vi "D3DM_comm.vi"() -> ()   [LabVIEW 2013]
uses:
  <vilib>/Native 3D Graph/xcontrol/3DPC_SurfacePlot.xctl
  <vilib>/Platform/NI_3dgraph.lvlib
panel:
  out "InRange":bool
  in  "3D Curve - Lorenz Attractor":refnum<k7>(container)
  in  "Simulation":bool
  in  "Least Dis":dbl=200.0
  in  "holder_length":dbl=87.37
  in  "Arm Angle Set":i32(slide)=1456 min=750 max=2150 step=1 scale=750.0..2150.0
  out "Title":string="      Distributed 3D Measurement Control Panel"
  in  "Log File Path":path=path "E:/Dropbox/StaredProject/Distributed3D/D3DM/raw_log.txt"
  in  "Port":u16=8899
  in  "Base Rotation Speed Set":i32(slide)=1471 min=1000 max=2000 step=1 scale=1000.0..2000.0
  in  "Command":string
  in  "Byte to Read(TCP)":i32=512
  out "Read Buffer":string
  out "help":string="1.Set the target Port number;\n2.Press \"Ready\" button to start acquiring data;\n3.Use arrow keys to control movement;\n4.Use the speed pointer slide to control speed;\n5.Use the Arm Angle slide to control arm;\n6.Press \"ESC\" to stop the car, 3D plot should be     finished automatically."
  in  "ArcStepThreshold":dbl=8000.0
  out "3D Graph":refnum<class "Base Datatype.lvclass">[](xcontrol)
  in  "Stop Button":bool
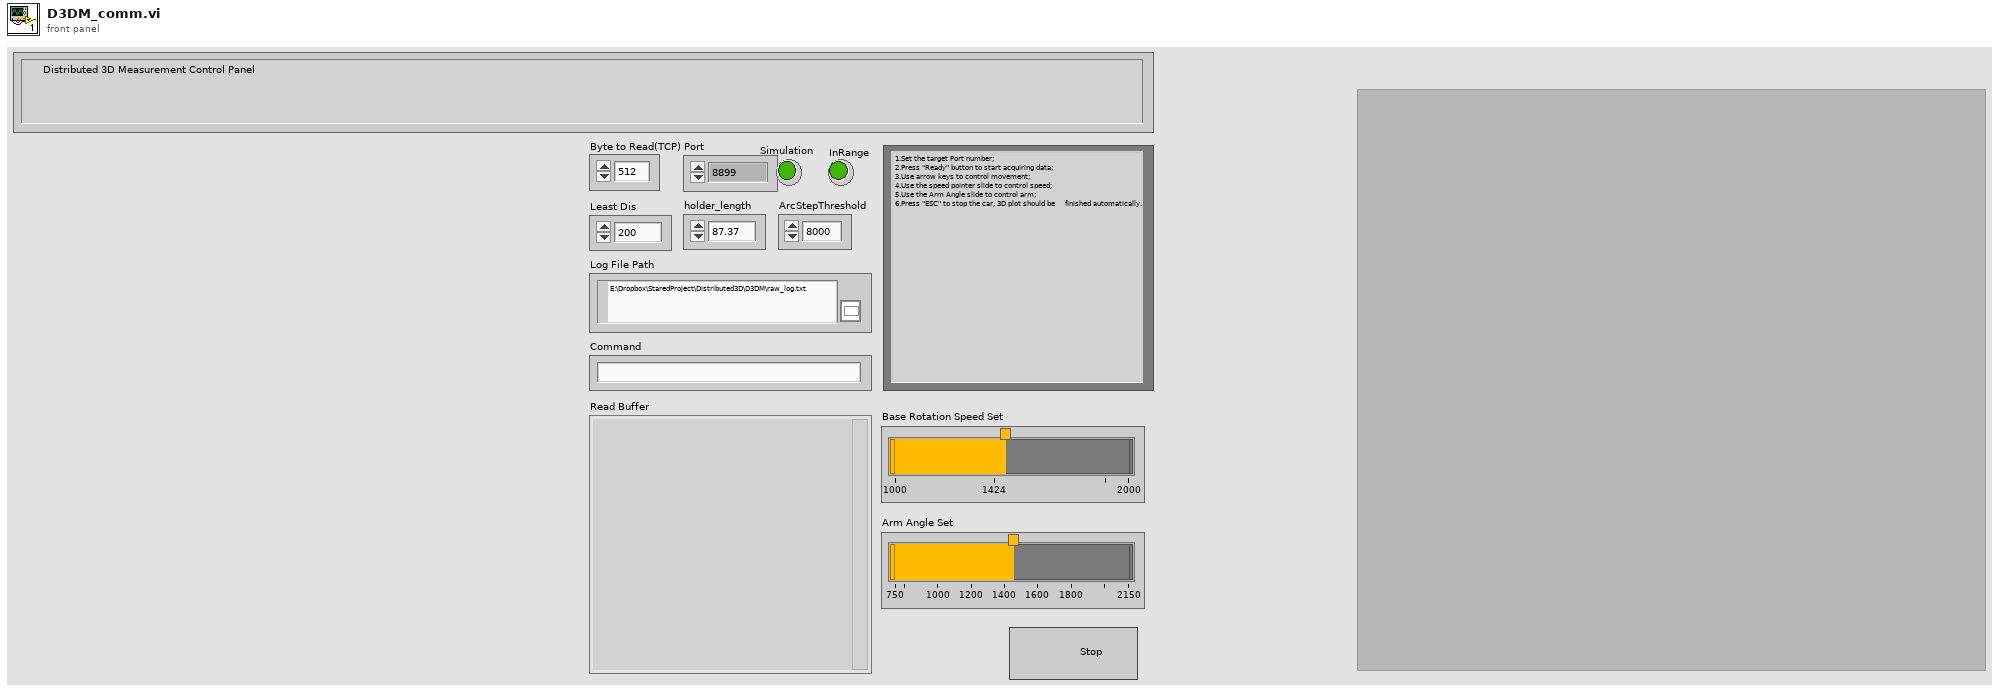
[diagram p1: front panel]
types:
  T1 = enum16{"open", "replace", "create", "open or create", "replace or create", "replace or create with confirmation"}
  T2 = typedef "eventvkey.ctl" = enum16{"ASCII", "Enter", "Return", "Shift", "Ctrl", "Alt", "Cmd", "Opt", "Caps", "NumLock", "Clear", "Break", "Up", "Down", "Left", "Right", "Insert", "Delete", "Home", "End", "PageUp", "PageDown", "Escape", "Help", "Pause", "ScrollLock", "F1", "F2", "F3", "F4", "F5", "F6", "F7", "F8", "F9", "F10", "F11", "F12", "F13", "F14", "F15", "F16", "F17", "F18", "F19", "F20", "F21", "F22", "F23", "F24", "Play", "VolumeUp", "VolumeDown", "Mute", "Two Byte Char"}
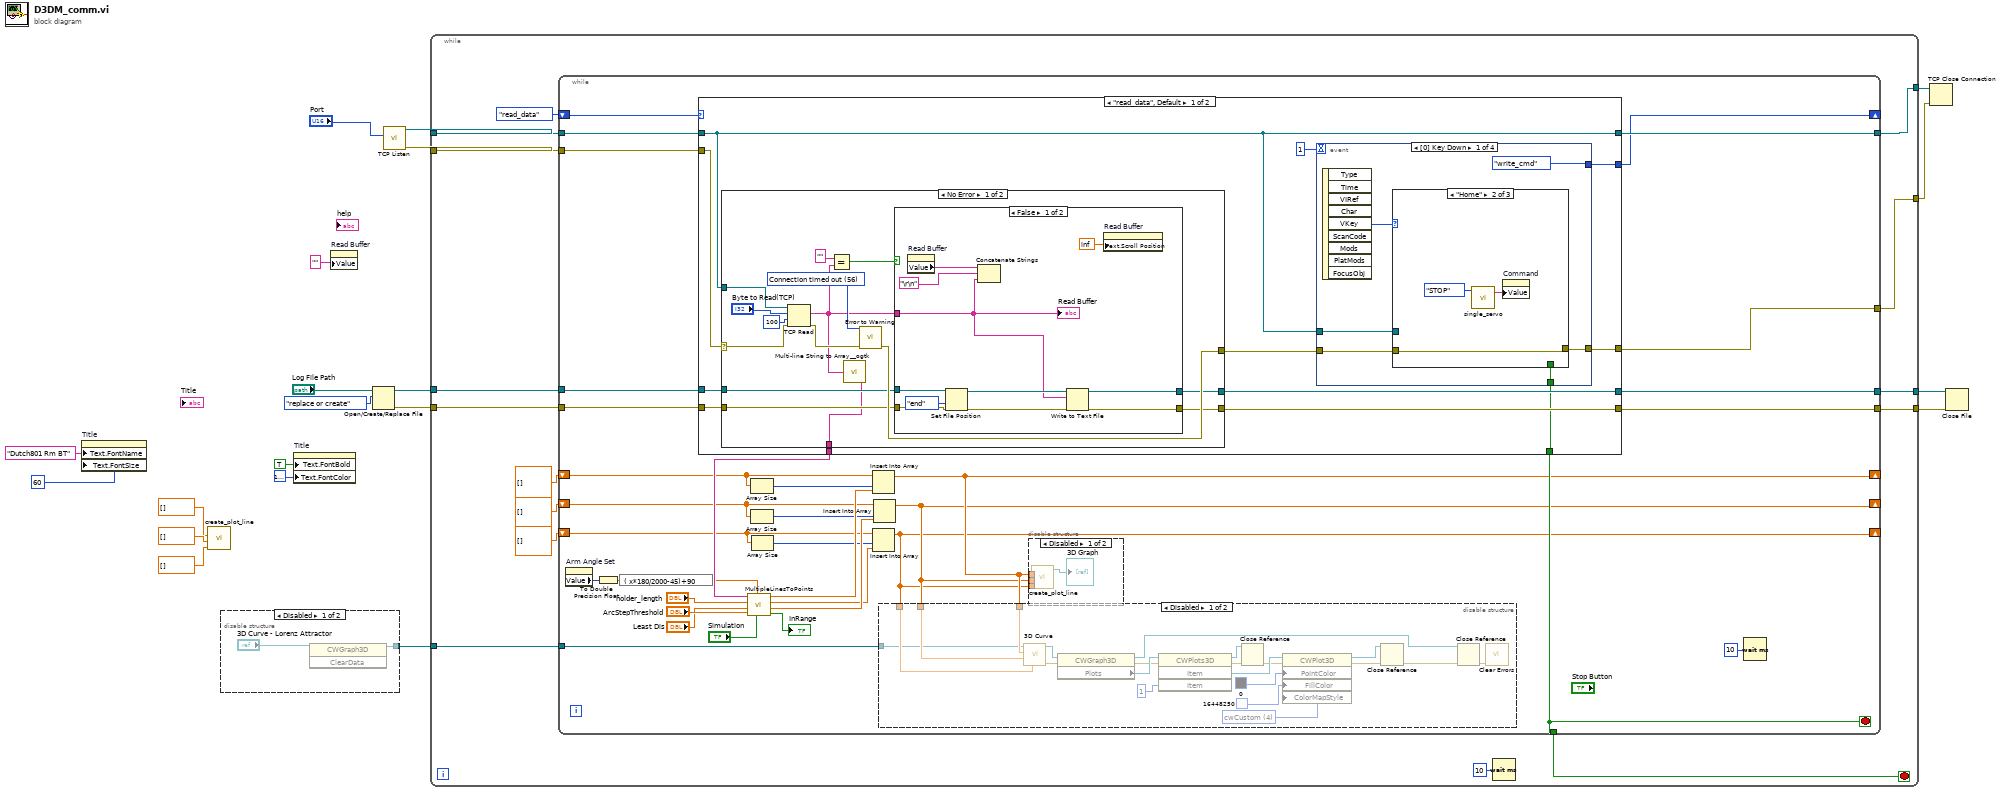
[diagram p0: block diagram]
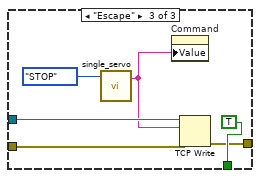
[diagram p6: hidden frame]
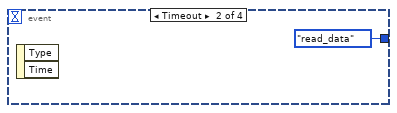
[diagram p7: hidden frame]
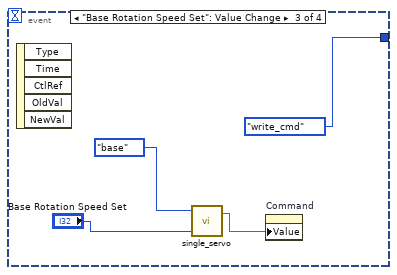
[diagram p8: hidden frame]
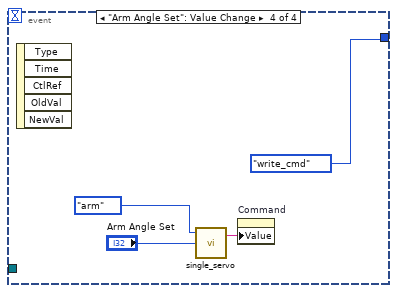
[diagram p9: hidden frame]
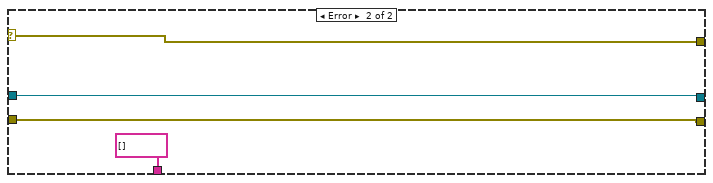
[diagram p11: hidden frame]
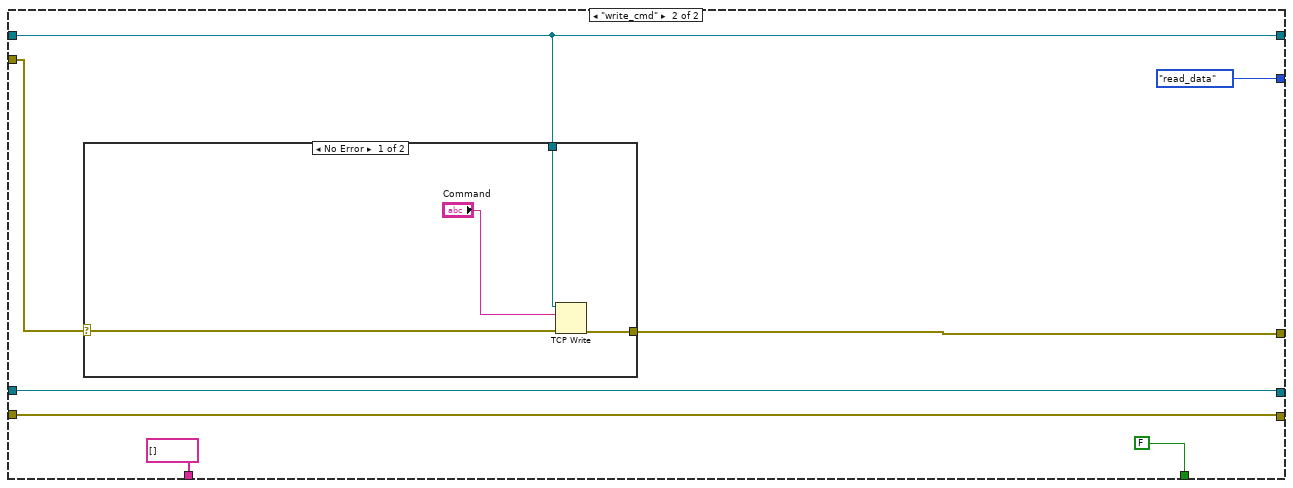
[diagram p12: hidden frame]
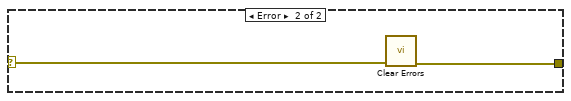
[diagram p13: hidden frame]
diagram:
  n1 = property on="Title" class="Str"("Text.FontName"="Dutch801 Rm BT" ("Text.Font:Name"), "Text.FontSize"=u32 60 ("Text.Font:Size")) -> ()  [unwired: 2 in, 2 out]
  n2 = call <vilib>:"create_plot_line.vi"("z vector"=dbl[] [], "y vector"=dbl[] [], "x vector"=dbl[] []) -> ()  [unwired: 8 in, 1 out]
  n3 = disable-structure shown="Disabled" {
    disable-tunnel: [w21 _] -> w1
    frame Disabled {
      n4 = invoke class="CWGraph3D" method="ClearData"(reference="3D Curve - Lorenz Attractor") -> (reference out=w21:refnum<k7>)  [unwired: 2 in, 2 out]
    }
    frame Enabled {
    }
  }
  n5 = property on="Title" class="Str"("Text.FontBold"=TRUE ("Text.Font:Bold"), "Text.FontColor"=u32 16777222) -> ()  [unwired: 2 in, 2 out]
  n6 = property on="Read Buffer" class="Str"("Value"="") -> ()  [unwired: 2 in, 2 out]
  n7 = Open/Create/Replace File(file path (use dialog)="Log File Path", operation (0:open)=T1."replace or create") -> (refnum out=w13:refnum<file>, error out=w12:errorcluster)  [unwired: 4 in, 1 out]
  n8 = call <vilib>:"TCP Listen.vi"("port"="Port") -> ("error out"=w18:errorcluster, "connection ID"=w19:refnum<k5>)  [unwired: 6 in, 3 out]
  n9 = while {
    tunnel: w19 -> [w35]
    tunnel: w18 -> [w34]
    tunnel: [w33] -> w17
    tunnel: [w32] -> w16
    tunnel: w13 -> [w31]
    tunnel: w12 -> [w30]
    tunnel: [w29] -> w11
    tunnel: [w28] -> w10
    tunnel: w1 -> [w27]
    stop <- w36 stop-if-true
    n10 = while {
      shift-right: [w61] -> _
      shift-left: enum16{"read_data", "write_cmd"}."read_data" ("RWstate") -> [w71]
      tunnel: w34 -> [w70]
      tunnel: w35 -> [w69]
      tunnel: [w64] -> w36
      tunnel: w31 -> [w68]
      tunnel: w30 -> [w67]
      tunnel: [w66] -> w29
      tunnel: [w65] -> w28
      tunnel: [w63] -> w33
      tunnel: [w62] -> w32
      shift-right: [w49] -> _
      shift-left: dbl[] [] -> [w56]
      shift-right: [w48] -> _
      shift-left: dbl[] [] -> [w52]
      shift-right: [w47] -> _
      shift-left: dbl[] [] -> [w51]
      tunnel: w27 -> [w43]
      stop <- w64 stop-if-true
      n11 = property on="Arm Angle Set" class="Slide (strict)"() -> ("Value"=w41:i32)  [unwired: 2 in, 2 out]
      n12 = To Double Precision Float(number=w41) -> (double precision float=w39:dbl)
      n13 = expression code="( x*180/2000-45)+90"(w39) -> (w40:dbl)
      n14 = case shown="\"read_data\", Default" w71 {
        tunnel: w70 -> [w108 w173]
        tunnel: w69 -> [w100 w168]
        tunnel: w68 -> [w107 w172]
        tunnel: w67 -> [w106 w171]
        tunnel: [w105 w172] -> w66
        tunnel: [w104 w171] -> w65
        tunnel: [w103 FALSE] -> w64
        tunnel: [w101 w170] -> w63
        tunnel: [w100 w168] -> w62
        tunnel: [w99 enum16{"read_data", "write_cmd"}."read_data" ("RWstate")] -> w61
        tunnel: [w97 string[] [] ("lines")] -> w57
        frame "read_data", Default {
          n15 = case shown="No Error" w108 {
            selector: w108 -> [w140 w165]
            tunnel: [w144 w165] -> w102
            tunnel: w100 -> [w141 _]
            tunnel: w107 -> [w139 w164]
            tunnel: w106 -> [w138 w163]
            tunnel: [w137 w164] -> w105
            tunnel: [w136 w163] -> w104
            tunnel: [w134 string[] [] ("lines")] -> w97
            frame No Error {
              w148 = 56 items=["No Error", "Argument Error", "Memory Full", "Out of Zone", "End of File", "File Already Open", "Generic File IO Error", "File Not Found", "File Permission Error", "Disk Full", "Duplicate Path", "Too Many Files Open", "Not Enabled", "Resource File Not Found", "Cannot Add Resource", "Resource Not Found", "Image Not Found", "Image Memory Error", "Pen Does Not Exist", "Config Bad Type", "Config Token Not Found", "Config Parse Error", "Config Memory Error", "Bad External Code Format", "Bad External Code Offset", "External Code Not Present", "Null Window", "Destroy Window Mixup", "Null Menu", "Print Aborted", "Bad Print Record", "Print Driver Error", "Windows Error During Print", "Memory Error During Print", "Print Dialog Error", "Generic Print Error", "Invalid Device Refnum", "Device Not Found", "Device Parameter Error", "Device Unit Error", "Can't Open Device", "Device Call Aborted", "Generic Error", "Cancelled By User", "Object ID Too Low", "Object ID Too High", "Object Not In Heap", "Unknown Heap", "Bad DefProc ID", "DefProc Not In Table", "Message Out Of Range", "Null Method", "Unknown Message", "Manager Call Not Supported", "Bad address", "Connection In progress", "Connection timed out", "Connection is already in progress", "Network attribute not supported", "Network error", "Address in use", "System out of memory", "Connection aborted", "Connection refused", "Connection is not connected", "Connection is already connected", "Connection closed", "Initialize error (interapplication manager)", "Bad occurrence", "Wait on unbound occurrence handler", "Occurrence queue overflow", "Bad path", "Semaphore not signaled", "Unrecognized type (interapplication manager)"] ("1st Error to Convert")
              n16 = TCP Read(connection ID=w141, bytes to read="Byte to Read(TCP)", error in (no error)=w140, 9:100) -> (data out=w135:string, error out=w147:errorcluster)  [unwired: 1 in, 1 out]
              n17 = Equal?(x="", y=w135) -> (x = y?=w143:bool)
              n18 = call <userlib>:"Multi-line String to Array__ogtk.vi"("string"=w135) -> ("lines"=w134:string[])
              n19 = call <vilib>:"Error to Warning.vi"("1st Error to Convert"=w148, "error in"=w147) -> ("warning out"=w144:errorcluster)  [unwired: 13 in]
              n20 = case shown="False" w143 {
                tunnel: w135 -> [w149 _]
                tunnel: w139 -> [w156 w161]
                tunnel: w138 -> [w155 w160]
                tunnel: [w151 w161] -> w137
                tunnel: [w150 w160] -> w136
                frame False {
                  n21 = property on="Read Buffer" class="Str"() -> ("Value"=w157:string)  [unwired: 2 in, 2 out]
                  n22 = Set File Position(refnum=w156, from (0:start)=enum16{"start", "end", "current"}."end", error in=w155) -> (refnum out=w154:refnum<file>, error out=w153:errorcluster)  [unwired: 1 in]
                  n23 = Concatenate Strings(w157, "\r\n", w149) -> ()  [unwired: 1 out]
                  n24 = Write to Text File(file (use dialog)=w154, text=w149, error in=w153) -> (refnum out=w151:refnum<file>, error out=w150:errorcluster)  [unwired: 1 in, 1 out]
                  n25 = property on="Read Buffer" class="Str"("Text.Scroll Position"=inf) -> ()  [unwired: 2 in, 2 out]
                  "Read Buffer" <- w149
                }
                frame True {
                }
              }
            }
            frame Error {
            }
          }
          n26 = event shown="[0] Key Down" {
            selector: _ -> [_ _ _ _]
            dyn-events: _ -> [_ _ _ _]
            timeout: 1 -> [_ _ _ _]
            tunnel: [enum16{"read_data", "write_cmd"}."write_cmd" ("RWstate") enum16{"read_data", "write_cmd"}."read_data" ("RWstate") enum16{"read_data", "write_cmd"}."write_cmd" ("RWstate") enum16{"read_data", "write_cmd"}."write_cmd" ("RWstate")] -> w99
            tunnel: [w113 _ _ _] -> w103
            tunnel: [w111 _ _ _] -> w101
            tunnel: w100 -> [w110 _ _ _]
            tunnel: w102 -> [w109 _ _ _]
            event Key Down {
              n27 = event-data() -> ("VKey"=w112:T2)  [unwired: 1 in, 8 out]
              n28 = case shown="\"Home\"" w112 {
                tunnel: [_ _ TRUE] -> w113
                tunnel: [w115 w118 w123] -> w111
                tunnel: w110 -> [_ _ w122]
                tunnel: w109 -> [w115 w118 w121]
                frame "ASCII", Default {
                }
                frame "Home" {
                  n29 = call "single_servo.vi"("ServoControl"=enum16{"STOP", "both", "arm", "base"}."STOP") -> ("cmd"=w116:string)  [unwired: 3 in]
                  n30 = property on="Command" class="Str"("Value"=w116) -> ()  [unwired: 2 in, 2 out]
                }
                frame "Escape" {
                  n31 = call "single_servo.vi"("ServoControl"=enum16{"STOP", "both", "arm", "base"}."STOP") -> ("cmd"=w119:string)  [unwired: 3 in]
                  n32 = property on="Command" class="Str"("Value"=w119) -> ()  [unwired: 2 in, 2 out]
                  n33 = TCP Write(connection ID=w122, data in=w119, error in (no error)=w121) -> (error out=w123:errorcluster)  [unwired: 1 in, 2 out]
                }
              }
            }
            event Timeout {
              n34 = event-data() -> ()  [unwired: 1 in, 2 out]
            }
            event "Base Rotation Speed Set": Value Change {
              n35 = event-data() -> ()  [unwired: 1 in, 5 out]
              n36 = call "single_servo.vi"("base_set"="Base Rotation Speed Set", "ServoControl"=enum16{"STOP", "both", "arm", "base"}."base") -> ("cmd"=w128:string)  [unwired: 2 in]
              n37 = property on="Command" class="Str"("Value"=w128) -> ()  [unwired: 2 in, 2 out]
            }
            event "Arm Angle Set": Value Change {
              n38 = event-data() -> ()  [unwired: 1 in, 5 out]
              n39 = call "single_servo.vi"("arm_set"="Arm Angle Set", "ServoControl"=enum16{"STOP", "both", "arm", "base"}."arm") -> ("cmd"=w132:string)  [unwired: 2 in]
              n40 = property on="Command" class="Str"("Value"=w132) -> ()  [unwired: 2 in, 2 out]
            }
          }
        }
        frame "write_cmd" {
          n41 = case shown="No Error" w173 {
            selector: w173 -> [w176 w178]
            tunnel: [w177 w179] -> w170
            tunnel: w168 -> [w175 _]
            frame No Error {
              n42 = TCP Write(connection ID=w175, data in="Command", error in (no error)=w176) -> (error out=w177:errorcluster)  [unwired: 1 in, 2 out]
            }
            frame Error {
              n43 = call <vilib>:"Clear Errors.vi"("error in (no error)"=w178) -> ("error out"=w179:errorcluster)  [unwired: 6 in]
            }
          }
        }
      }
      n44 = call "MultipleLinesToPoints.vi"("Sim"="Simulation", "theta2_open"=w40, "Arc Threshold"="ArcStepThreshold", "Least Dis"="Least Dis", "holder_length"="holder_length", "lines"=w57) -> ("InRange"=→"InRange":bool, "y"=w59:dbl[], "z"=w58:dbl[], "x"=w60:dbl[])
      n45 = Array Size(array=w56) -> (size(s)=w55:i32)
      n46 = Array Size(array=w52) -> (size(s)=w54:i32)
      n47 = Array Size(array=w51) -> (size(s)=w53:i32)
      n48 = Insert Into Array(array=w56, index=w55, new element=w60) -> (w49:dbl[])
      n49 = Insert Into Array(array=w51, index=w53, new element=w58) -> (w47:dbl[])
      n50 = Insert Into Array(array=w52, index=w54, new element=w59) -> (w48:dbl[])
      n51 = disable-structure shown="Disabled" {
        disable-tunnel: w49 -> [w78 _]
        disable-tunnel: w48 -> [w77 _]
        disable-tunnel: w47 -> [w76 _]
        disable-tunnel: w43 -> [w72 _]
        frame Disabled {
          w73 = 4 items=["cwNone", "cwShaded", "cwColorSpectrum", "cwGrayScale", "cwCustom"] ("ColorMapStyle")
          n52 = call <vilib>:"3D Curve.vi"("z vector"=w76, "y vector"=w77, "x vector"=w78, "3D graph"=w72) -> ("error out"=w90:errorcluster, "3D graph out"=w89:refnum<k7>)  [unwired: 6 in]
          n53 = property class="CWGraph3D"(reference=w89, error in=w90) -> (reference out=w80:refnum<k7>, error out=w88:errorcluster, "Plots"=w92:refnum<k7>)
          n54 = invoke class="CWPlots3D" method="Item"(reference=w92, error in=w88, "Item"=1) -> (reference out=w86:refnum<k7>, error out=w87:errorcluster, "Item"=w91:refnum<k7>)  [unwired: 1 in, 1 out]
          n55 = Close Reference(reference=w86, error in (no error)=w87) -> (error out=w85:errorcluster)
          n56 = property class="CWPlot3D"(reference=w91, error in=w85, "PointColor"=u32 0, "FillColor"=u32 16448250, "ColorMapStyle"=w73) -> (reference out=w83:refnum<k7>, error out=w84:errorcluster)
          n57 = Close Reference(reference=w83, error in (no error)=w84) -> (error out=w81:errorcluster)
          n58 = Close Reference(reference=w80, error in (no error)=w81) -> (error out=w82:errorcluster)
          n59 = call <vilib>:"Clear Errors.vi"("error in (no error)"=w82) -> ()  [unwired: 6 in, 1 out]
        }
        frame Enabled {
        }
      }
      n60 = disable-structure shown="Disabled" {
        disable-tunnel: w49 -> [w95 _]
        disable-tunnel: w48 -> [w94 _]
        disable-tunnel: w47 -> [w93 _]
        frame Disabled {
          n61 = call <vilib>:"create_plot_line.vi"("z vector"=w93, "y vector"=w94, "x vector"=w95) -> ("plots out"=→"3D Graph":refnum<class "Base Datatype.lvclass">[])  [unwired: 8 in]
        }
        frame Enabled {
        }
      }
      n62 = Wait (ms)(milliseconds to wait=u32 10) -> ()  [unwired: 1 out]
    }
    n63 = Wait (ms)(milliseconds to wait=u32 10) -> ()  [unwired: 1 out]
  }
  n64 = TCP Close Connection(connection ID=w16, error in (no error)=w17) -> ()  [unwired: 1 in, 2 out]
  n65 = Close File(refnum=w11, error in=w10) -> ()  [unwired: 2 out]
